vi "HallMeasurementTcpSample.vi"() -> ()   [LabVIEW 2017]
doc: "ホール測定PC用TCP通信サンプル"
uses:
  SubVI/HallMeasurementStatus.ctl
  SubVI/TcpCommunicationClientCMD.ctl
panel:
  out "TcpOK?":bool
  in  "Start":bool
  in  "DataFilePath":path=path "Test"
  out "SettingFilePath":path
  out "SampleName":string
  in  "Status":T1
  out "ReadData":string
  in  "Send Data":string
  in  "Send":bool
  in  "ポート":u16=8501
  in  "中央PCアドレス":string="localhost"
  in  "停止":bool
  # "1. 「中央PCアドレス」にIPアドレスを入力します。例：192.168.0.0\n　同じPCで実行する場合は　localhost　のまま実行\n\n2. マネージャーPC用TCP通信サンプル（ManagerTcpSample.vi）を実行します。\n\n3. このVIを実行します。\n　ManagerTcpSample.viにこちらのIPアドレスが表示されます。\n\n4. ManagerTcpSample.viのホール測定PCアドレスにこちらのアドレスを入力します。\n\n5. ManagerTcpSample.viのボタンを押すと対応するコマンドが送られます。\n\n6. 受信したコマンドに応じて自動で返信を送信します。\n\n7. コマンドに対応してStatusやFilePath、StartやOKのLEDが変化します。\n\n8. 停止時はこちらのソフトを先に止めます。"
  # "ホール測定PC用TCP通信サンプル"
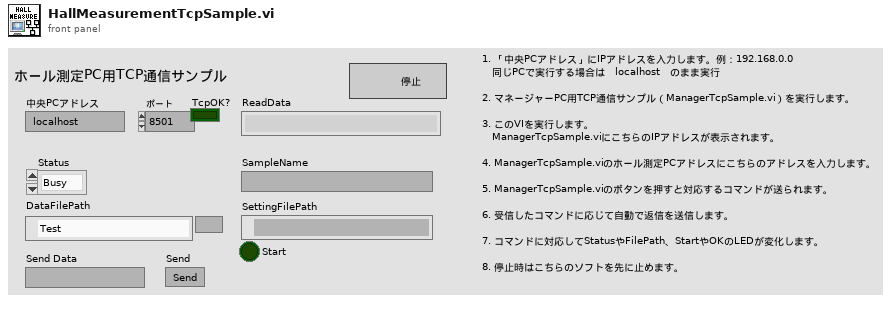
[diagram p1: front panel]
types:
  T1 = typedef "HallMeasurementStatus.ctl" = enum16{"Busy", "Ready", "Done", "Error"}
  T2 = typedef "TcpCommunicationClientCMD.ctl" = enum16{"Read", "Write", "Close"}
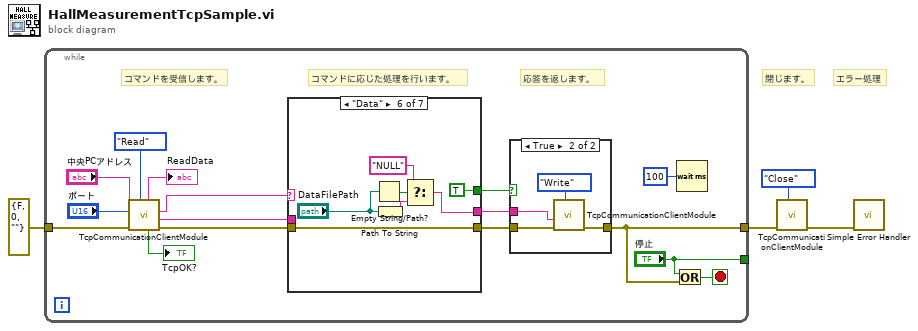
[diagram p0: block diagram]
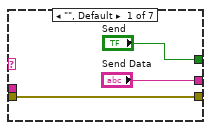
[diagram p3: hidden frame]
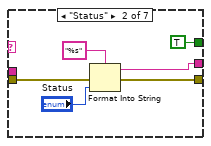
[diagram p4: hidden frame]
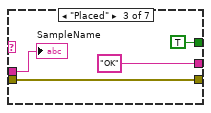
[diagram p5: hidden frame]
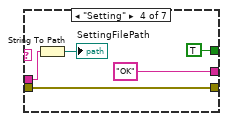
[diagram p6: hidden frame]
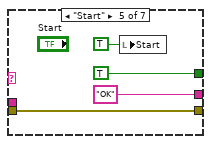
[diagram p7: hidden frame]
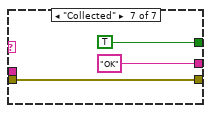
[diagram p8: hidden frame]
diagram:
  # "エラー処理"
  # "閉じます。"
  n1 = while {
    tunnel: ["停止"] -> _
    tunnel: [w9] -> w2
    tunnel: errorcluster {"status"=FALSE, "code"=0, "source"=""} ("エラー入力（エラーなし）") -> [w16]
    stop <- w20 stop-if-true
    # "応答を返します。"
    # "コマンドに応じた処理を行います。"
    # "コマンドを受信します。"
    n2 = call "TcpCommunicationClientModule.vi"("TcpCommunicationClientCMD"=TcpCommunicationClientCMD."Read", "エラー入力（エラーなし）"=w16, "ポート"="ポート", "アドレス"="中央PCアドレス") -> ("エラー出力"=w18:errorcluster, "Data"=w6:string, "Command"=w7:string, "TcpOK?"=→"TcpOK?":bool, "ReadData"=→"ReadData":string)  [unwired: 3 in]
    n3 = case shown="\"Data\"" w7 {
      tunnel: w6 -> [_ _ w35 w40 _ _ _]
      tunnel: ["Send Data" w32 "OK" ("Send Data") "OK" ("Send Data") "OK" ("Send Data") w49 "OK" ("Send Data")] -> w11
      tunnel: ["Send" TRUE ("Send") TRUE ("Send") TRUE ("Send") TRUE ("Send") TRUE ("Send") TRUE ("Send")] -> w12
      tunnel: w18 -> [w26 w30 w37 w42 w46 w53 w56]
      tunnel: [w26 w29 w37 w42 w46 w53 w56] -> w10
      frame "", Default {
      }
      frame "Status" {
        n4 = Format Into String(format string="%s" ("形式文字列"), error in=w30, "Status") -> (resulting string=w32:string, error out=w29:errorcluster)  [unwired: 1 in]
      }
      frame "Placed" {
        "SampleName" <- w35
      }
      frame "Setting" {
        n5 = String To Path(string=w40) -> (path=→"SettingFilePath":path)
      }
      frame "Start" {
        n6 = local write "Start"(TRUE) -> ()
      }
      frame "Data" {
        n7 = Empty String/Path?(string/path="DataFilePath") -> (empty?=w51:bool)
        n8 = Path To String(path="DataFilePath") -> (string=w50:string)
        n9 = Select(t="NULL", s=w51, f=w50) -> (s? t:f=w49:string)
      }
      frame "Collected" {
      }
    }
    n10 = case shown="TRUE" w12 {
      tunnel: w10 -> [w21 w25]
      tunnel: [w21 w24] -> w9
      tunnel: w11 -> [_ w22]
      frame False {
      }
      frame True {
        n11 = call "TcpCommunicationClientModule.vi"("TcpCommunicationClientCMD"=TcpCommunicationClientCMD."Write", "エラー入力（エラーなし）"=w25, "WriteData"=w22) -> ("エラー出力"=w24:errorcluster)  [unwired: 4 in, 4 out]
      }
    }
    n12 = Or(x="停止", y=w9) -> (x .or. y?=w20:bool)
    n13 = Wait (ms)(milliseconds to wait=u32 100 ("ミリ秒待機時間")) -> ()  [unwired: 1 out]
  }
  n14 = call "TcpCommunicationClientModule.vi"("TcpCommunicationClientCMD"=TcpCommunicationClientCMD."Close", "エラー入力（エラーなし）"=w2) -> ("エラー出力"=w1:errorcluster)  [unwired: 5 in, 4 out]
  n15 = call <vilib>:"Simple Error Handler.vi"("error in (no error)"=w1) -> ()  [unwired: 1 in, 8 out]
